vi "Release_Save.vi"(8 "Error In":errorcluster, 11 "Queue Cluster":T1) -> ()   [LabVIEW 2021, in "Queues.lvlib"]
doc: "This VI is used to destroy the queues, notifiers, user events of the Save VI."
uses:
  Queues.lvlib
  Tipski Definicii/Save_Sostojbi.ctl
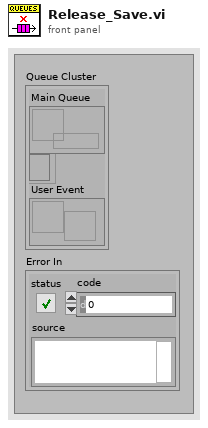
[diagram p1: front panel]
types:
  T1 = cluster{"Main Queue":refnum<queue>, "ER Refnum":refnum<event-registration>, "User Event":refnum<user-event>}
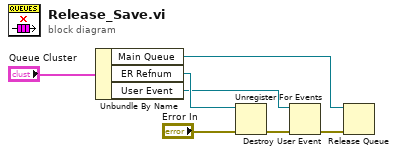
[diagram p0: block diagram]
diagram:
  n1 = Unbundle By Name("Queue Cluster") -> ("Main Queue"=w1:refnum<queue>, "ER Refnum"=w6:refnum<event-registration>, "User Event"=w3:refnum<user-event>)
  n2 = Unregister For Events(event registration refnum=w6, error in="Error In") -> (error out=w4:errorcluster)
  n3 = Destroy User Event(user event=w3, error in=w4) -> (error out=w2:errorcluster)
  n4 = Release Queue(queue=w1, error in (no error)=w2) -> ()  [unwired: 1 in, 3 out]
